vi "DraggingDresser.vi"() -> ()   [LabVIEW 2015]
panel:
  out "Force":dbl[](array[numeric])
  out "Angle for Minimum Force":i32 format="%.1f"
  in  "Coefficient of Kinetic Friction":dbl format="%.1f"
  out "Waveform Graph":dbl[](graph)
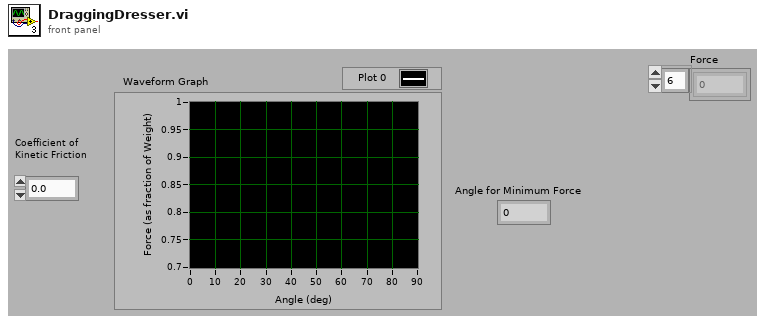
[diagram p1: front panel]
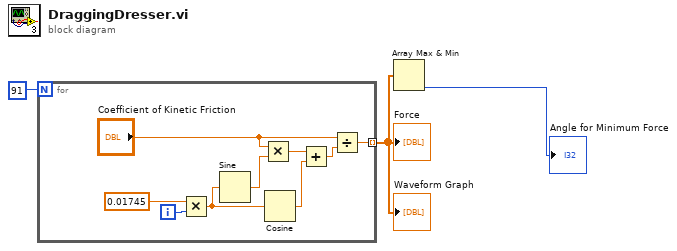
[diagram p0: block diagram]
diagram:
  n1 = for {
    N: 91 -> [_]
    tunnel: [w4] -> w2 mode=indexing
    i -> [w12]
    n2 = Multiply(x=0.01745, y=w12) -> (x*y=w10:dbl)
    n3 = Sine(x=w10) -> (sin(x)=w9:dbl)
    n4 = Multiply(x="Coefficient of Kinetic Friction", y=w9) -> (x*y=w8:dbl)
    n5 = Cosine(x=w10) -> (cos(x)=w7:dbl)
    n6 = Add(x=w8, y=w7) -> (x+y=w5:dbl)
    n7 = Divide(x="Coefficient of Kinetic Friction", y=w5) -> (x/y=w4:dbl)
  }
  "Force" <- w2
  "Waveform Graph" <- w2
  n8 = Array Max & Min(array=w2) -> (min index (indices)=→"Angle for Minimum Force":i32)  [unwired: 3 out]
